vi "Get Target Reference.vi"(6 "error in":errorcluster, 8 "Targets":refnum<vi>[](array[refnum]), 9 "Target":string="RT Target") -> (0 "error out":errorcluster, 1 "Found?":bool, 2 "Targets out":refnum<vi>[](array[refnum]), 3 "RT Target Refnum":refnum<vi>)   [LabVIEW 2010]
doc: "Returns the reference of \"RT Target\" from an array of targets"
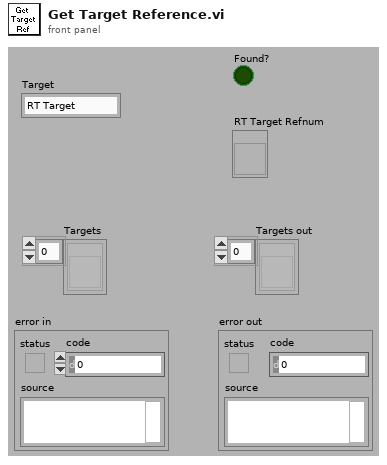
[diagram p1: front panel]
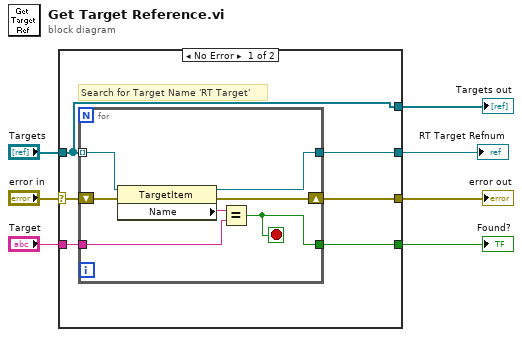
[diagram p0: block diagram]
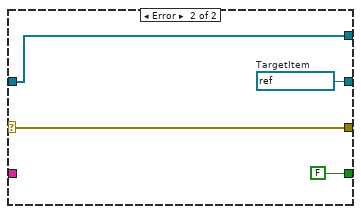
[diagram p2: hidden frame]
diagram:
  n1 = case shown="No Error" "error in" {
    selector: "error in" -> [w11 w24]
    tunnel: [w13 w23] -> w7
    tunnel: [w12 w24] -> w6
    tunnel: "Targets" -> [w10 w22]
    tunnel: [w10 w22] -> w3
    tunnel: "Target" -> [w9 _]
    tunnel: [w8 FALSE] -> w1
    frame No Error {
      # "Search for Target Name 'RT Target'"
      n2 = for {
        tunnel: w10 -> [w17] mode=indexing
        tunnel: [w16] -> w13
        shift-right: [w20] -> w12
        shift-left: w11 -> [w19]
        tunnel: w9 -> [w15]
        tunnel: [w14] -> w8
        stop <- w14 stop-if-true
        n3 = property class="TargetItem"(reference=w17, error in=w19) -> (reference out=w16:refnum<vi>, error out=w20:errorcluster, "Name"=w18:string)
        n4 = Equal?(x=w18, y=w15) -> (x = y?=w14:bool)
      }
    }
    frame Error {
      w23 = refnum<vi> refnum  # TargetItem
    }
  }
  "error out" <- w6
  "RT Target Refnum" <- w7
  "Targets out" <- w3
  "Found?" <- w1
